vi "SimpleJsonNQueryFromFile.vi"(8 "error in":errorcluster, 10 "Lookups":string[](array[string]), 11 "Json File":path) -> (0 "error out":errorcluster, 2 "Value As Numeric":dbl[](array[numeric]), 3 "Values As String":string[](array[string]))   [LabVIEW 2020]
doc: "Given a json file, extract values at the specified lookup strings ('keys')"
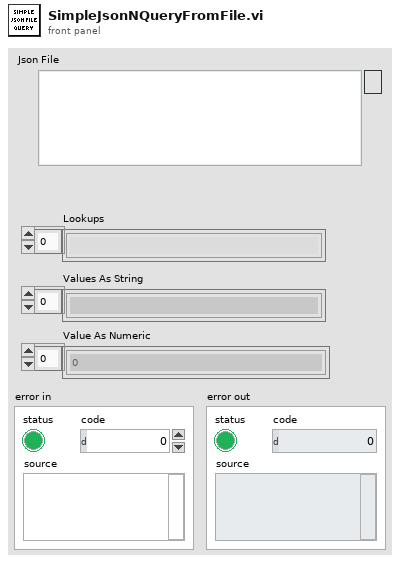
[diagram p1: front panel]
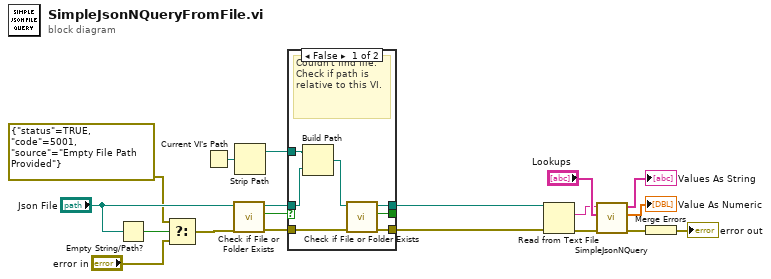
[diagram p0: block diagram]
diagram:
  n1 = Empty String/Path?(string/path="Json File") -> (empty?=w4:bool)
  n2 = Select(t=errorcluster {"status"=TRUE, "code"=5001, "source"="Empty File Path Provided"}, s=w4, f="error in") -> (s? t:f=w2:errorcluster)
  n3 = Current VI's Path() -> (path=w11:path)
  n4 = call <vilib>:"Check if File or Folder Exists.vi"("error in (no error)"=w2, "path"="Json File") -> ("error out"=w8:errorcluster, "file or folder exists?"=w10:bool, "dup path"=w9:path)  [unwired: 7 in]
  n5 = Strip Path(path=w11) -> (stripped path=w12:path)  [unwired: 1 out]
  n6 = case shown="False" w10 {
    selector: w10 -> [_ w27]
    tunnel: [w24 w29] -> w5
    tunnel: w8 -> [w26 w29]
    tunnel: [w25 w28] -> w6
    tunnel: w9 -> [w21 w28]
    tunnel: [w23 w27] -> _
    tunnel: w12 -> [w20 _]
    frame False {
      # "Couldn't find file.\nCheck if path is relative to this VI."
      n7 = Build Path(base path=w20, name or relative path=w21) -> (appended path=w22:path)
      n8 = call <vilib>:"Check if File or Folder Exists.vi"("error in (no error)"=w26, "path"=w22) -> ("error out"=w24:errorcluster, "file or folder exists?"=w23:bool, "dup path"=w25:path)  [unwired: 7 in]
    }
    frame True {
      # "Found file,\nNo worries"
    }
  }
  n9 = Read from Text File(file (use dialog)=w6, error in=w5) -> (text=w14:string, error out=w13:errorcluster)  [unwired: 2 in, 2 out]
  n10 = call "SimpleJsonNQuery.vi"("error in"=w13, "Lookups"="Lookups", "JsonString"=w14) -> ("error out"=w17:errorcluster, "Value As Numeric"=→"Value As Numeric":dbl[], "Values As String"=→"Values As String":string[])  [unwired: 6 in]
  n11 = Merge Errors(w17) -> (→"error out":errorcluster)
